vi "Set Addressable Endpoints.vi"(8 "error in (no error)":errorcluster, 10 "Addressable Endpoints":string[](array[string]), 11 "Hardware Ref in":T1 format="%.0x") -> (0 "error out":errorcluster, 3 "Hardware Ref out":T1 format="%.0x")   [LabVIEW 2017, in "Routing and Faulting Hardware API.lvlib"]
uses:
  Routing and Faulting Hardware API.lvlib
  <vilib>/NI Veristand/Custom Device API/Custom Device Item Ref.ctl
  Routing and Faulting Hardware API Constants.vi
  <vilib>/NI Veristand/Custom Device API/Set Item Property (String Array).vi
  <vilib>/NI Veristand/Custom Device API/Custom Device API.lvlib
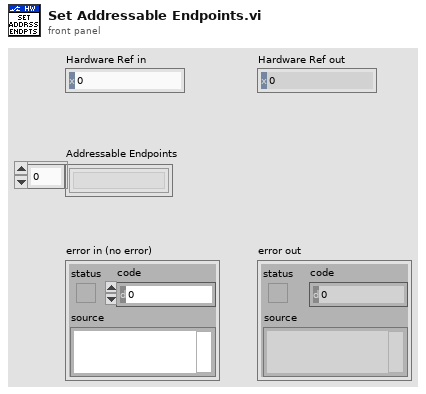
[diagram p1: front panel]
types:
  T1 = typedef "Custom Device API.lvlib/Custom Device Item Ref.ctl" = u64
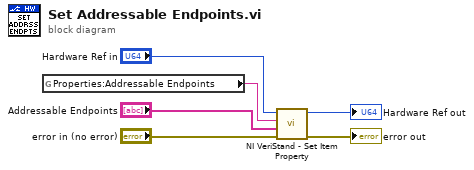
[diagram p0: block diagram]
diagram:
  n1 = global read "Routing and Faulting Hardware API Constants.vi" "Properties:Addressable Endpoints"() -> (w1:string)
  n2 = call-poly <vilib>:"NI VeriStand - Set Item Property.vi"("error in (no error)"="error in (no error)", "Value"="Addressable Endpoints", "Property Name"=w1, "Item Ref in"="Hardware Ref in") -> ("error out"=→"error out":errorcluster, "Item Ref out"=→"Hardware Ref out":T1)  [unwired: 5 in, 1 out]
